vi "2.while-loop.vi"() -> ()   [LabVIEW 2010]
panel:
  out "Loop-Iteration":dbl
  in  "stop":bool
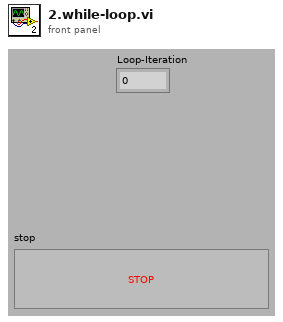
[diagram p1: front panel]
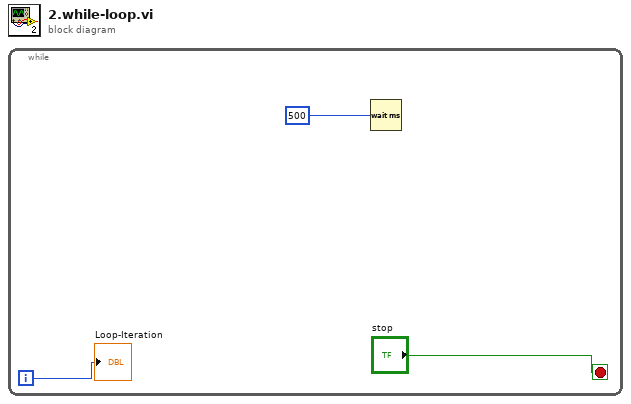
[diagram p0: block diagram]
diagram:
  n1 = while {
    i -> [w2]
    stop <- "stop" stop-if-true
    n2 = Wait (ms)(milliseconds to wait=500) -> ()  [unwired: 1 out]
    "Loop-Iteration" <- w2
  }
